vi "PathPlanner_GoalEndState_FromJSON.vi"(11 "JSON String":string) -> (0 "Exists":bool, 3 "GoalEndState":T1={"Velocity"=0.0, "Rotation"={"VALUE"=0.0, "COS"=1.0, "SIN"=0.0}} {"Rotation"."SIN" format="%13.4f"; "Rotation"."COS" format="%13.4f"; "Rotation"."VALUE" format="%13.4f"})   [LabVIEW 2019, in "PathPlanner24.lvlib"]
doc: "Create a goal end state from json\n\nInputs: \n -- JSON String - string - string to parse for GoalEndState\n\nOutputs:\n -- GoalEndState - cluster - The goal end state defined by the given json. If not found, default is returned.\n -- exists - boolean - TRUE if GoalEndState was found and parsed in the JSON string."
uses:
  PathPlanner24.lvlib
  TypeDef/PathPlannerGoalEndState.ctl
  <vilib>/Rock Robotics/WPI/ThirdParty/JAS_Junk/TrajLib/TypeDef/ROTATION2D.ctl
  <vilib>/Rock Robotics/WPI/ThirdParty/JAS_Junk/TrajLib/Conv_Deg_Radians.vi
  <vilib>/Rock Robotics/WPI/ThirdParty/JAS_Junk/TrajLib/Rotation2d_CreateAngle.vi
  <vilib>/Rock Robotics/WPI/ThirdParty/JAS_Junk/TrajLib/Trajectory_Library.lvlib
panel:
  in  "goalEndstate":cluster{"velocity":dbl, "rotation":dbl}
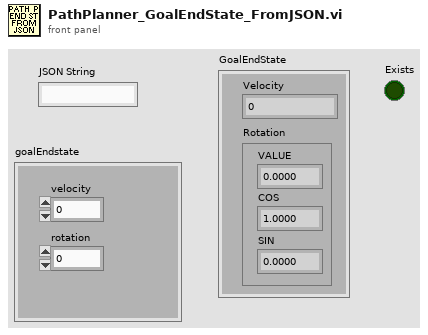
[diagram p1: front panel]
types:
  T1 = typedef "PathPlanner24.lvlib/PathPlannerGoalEndState.ctl" = cluster{"Velocity":dbl, "Rotation":T2}
  T2 = typedef "Trajectory_Library.lvlib/ROTATION2D.ctl" = cluster{"VALUE":dbl, "COS":dbl, "SIN":dbl}
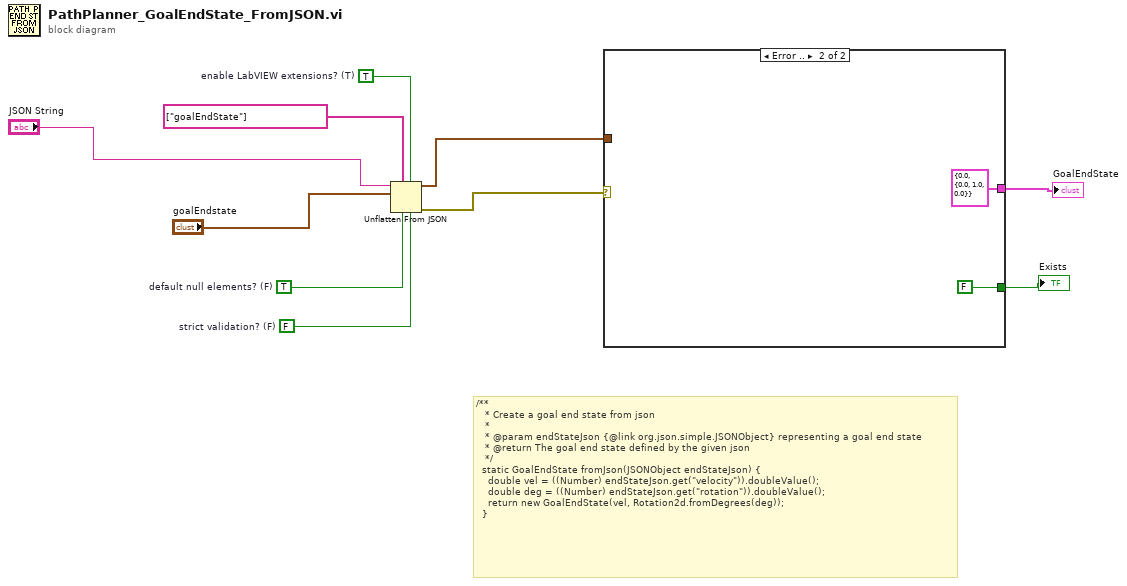
[diagram p0: block diagram]
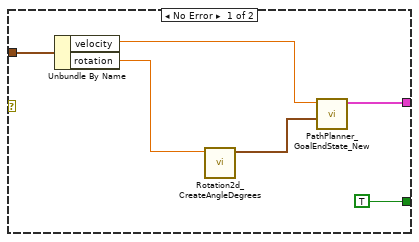
[diagram p2: hidden frame]
diagram:
  w7 = FALSE  # strict validation? (F)
  w8 = TRUE  # default null elements? (F)
  w9 = TRUE  # enable LabVIEW extensions? (T)
  # "/**\n   * Create a goal end state from json\n   *\n   * @param endStateJson {@link org.json.simple.JSONObject} representing a goal end state\n   * @return The goal end state defined by the given json\n   */\n  static GoalEndState fromJson(JSONObject endStateJson) {\n    double vel = ((Number) endStateJson.get(\"velocity\")).doubleValue();\n    double deg = ((Number) endStateJson.get(\"rotation\")).doubleValue();\n    return new GoalEndState(vel, Rotation2d.fromDegrees(deg));\n  }"
  n1 = Unflatten From JSON(path=string[] ["goalEndState"] ("path 2"), enable LabVIEW extensions? (T)=w9, JSON string="JSON String", type and defaults="goalEndstate", default null elements? (F)=w8, strict validation? (F)=w7) -> (value=w5:cluster{"velocity":dbl, "rotation":dbl}, error out=w6:errorcluster)  [unwired: 1 in]
  n2 = case shown="Error .." w6 {
    tunnel: w5 -> [w16 _]
    tunnel: [TRUE FALSE] -> w4
    tunnel: [w11 T1 {"Velocity"=0.0, "Rotation"={"VALUE"=0.0, "COS"=1.0, "SIN"=0.0}} ("GoalEndState")] -> w1
    frame No Error {
      n3 = Unbundle By Name(w16) -> ("velocity"=w14:dbl, "rotation"=w12:dbl)
      n4 = call <vilib>:"Rotation2d_CreateAngleDegrees.vi"("Angle_Degrees"=w12) -> ("ROTATION"=w13:T2)  [unwired: 10 in]
      n5 = call "PathPlanner_GoalEndState_New.vi"("Rotation"=w13, "Velocity"=w14) -> ("GoalEndState"=w11:T1)  [unwired: 9 in]
    }
    frame Error {
    }
  }
  "GoalEndState" <- w1
  "Exists" <- w4
